vi "test bindata forth and back.vi"() -> ()   [LabVIEW 2018, in "LV-Julia_ZMQ-Roundtrip_lib.lvlib"]
uses:
  LV-Julia_ZMQ-Roundtrip_lib.lvlib
  05036e79-a137-49d8-b8bd-98c2707dfc19.vi
  d20d9b8d-18a0-4bcc-837d-245d5138e077.vi
  acfd4be8-0c55-499e-a24a-58fc6a9364d6.vi
  edd4ba47-7688-445c-9fb9-34873410a5b9.vi
  05036e79-a137-49d8-b8bd-98c2707dfc19.vi/236d3e0c-60a7-4ae5-9bc9-0ff41b983f05.vi
  05036e79-a137-49d8-b8bd-98c2707dfc19.vi/b449f9df-ee8d-489b-9487-897c21ba14eb.vi
  05036e79-a137-49d8-b8bd-98c2707dfc19.vi/e7b7674e-094d-4356-9454-cca6775f0358.vi
  05036e79-a137-49d8-b8bd-98c2707dfc19.vi/025d52f7-3b03-4309-bff2-4ec84fc3d60c.vi
  d20d9b8d-18a0-4bcc-837d-245d5138e077.vi/212a36f8-8f57-49c9-9677-432581b68510.vi
  d20d9b8d-18a0-4bcc-837d-245d5138e077.vi/69652d2b-db18-4aab-bd2f-35078bef0426.vi
  d20d9b8d-18a0-4bcc-837d-245d5138e077.vi/4772bca8-5d3a-4f2a-8bbf-c07de0696f94.vi
  d20d9b8d-18a0-4bcc-837d-245d5138e077.vi/7139aa7f-98bf-4369-975b-4bd5deaf00da.vi
  acfd4be8-0c55-499e-a24a-58fc6a9364d6.vi/b7780163-44f5-4435-ad3c-f5928cad1e22.vi
  acfd4be8-0c55-499e-a24a-58fc6a9364d6.vi/63841309-fb5d-4205-a56b-05074a2af6c9.vi
  edd4ba47-7688-445c-9fb9-34873410a5b9.vi/2b4cb753-bccd-455e-b921-2800034f5550.vi
  edd4ba47-7688-445c-9fb9-34873410a5b9.vi/9d483ba0-a828-48f7-8b88-1ec263ae9c55.vi
  05036e79-a137-49d8-b8bd-98c2707dfc19.vi/b449f9df-ee8d-489b-9487-897c21ba14eb.vi/9a929507-b059-4abd-9ed4-ef53a005ff63.vi
  05036e79-a137-49d8-b8bd-98c2707dfc19.vi/e7b7674e-094d-4356-9454-cca6775f0358.vi/ad73f5ce-7658-473b-b9fc-fac91a92da1e.vi
  05036e79-a137-49d8-b8bd-98c2707dfc19.vi/025d52f7-3b03-4309-bff2-4ec84fc3d60c.vi/5d27c3aa-c82a-4d9f-96ad-8781e4a71ba1.vi
  d20d9b8d-18a0-4bcc-837d-245d5138e077.vi/69652d2b-db18-4aab-bd2f-35078bef0426.vi/dfcf8de0-7860-4713-ab77-0e8f714dde10.vi
  d20d9b8d-18a0-4bcc-837d-245d5138e077.vi/4772bca8-5d3a-4f2a-8bbf-c07de0696f94.vi/e532232b-f4b6-4bbd-a5e7-664623875ae8.vi
  d20d9b8d-18a0-4bcc-837d-245d5138e077.vi/7139aa7f-98bf-4369-975b-4bd5deaf00da.vi/7a16f954-d622-4be0-bb4d-b4bfb8ef0f01.vi
  05036e79-a137-49d8-b8bd-98c2707dfc19.vi/b449f9df-ee8d-489b-9487-897c21ba14eb.vi/9a929507-b059-4abd-9ed4-ef53a005ff63.vi/47391a1c-e85f-44cf-90f5-ee97f4b4554e.vi
  05036e79-a137-49d8-b8bd-98c2707dfc19.vi/e7b7674e-094d-4356-9454-cca6775f0358.vi/ad73f5ce-7658-473b-b9fc-fac91a92da1e.vi/6213ee20-5898-4e73-9fb0-a99b3c67ea96.vi
  05036e79-a137-49d8-b8bd-98c2707dfc19.vi/025d52f7-3b03-4309-bff2-4ec84fc3d60c.vi/5d27c3aa-c82a-4d9f-96ad-8781e4a71ba1.vi/cb9fe9ca-b60f-4580-8939-faeac5c9a8ca.vi
  d20d9b8d-18a0-4bcc-837d-245d5138e077.vi/69652d2b-db18-4aab-bd2f-35078bef0426.vi/dfcf8de0-7860-4713-ab77-0e8f714dde10.vi/9577cbac-8520-44d1-a8fc-fc5a580fd613.vi
  d20d9b8d-18a0-4bcc-837d-245d5138e077.vi/4772bca8-5d3a-4f2a-8bbf-c07de0696f94.vi/e532232b-f4b6-4bbd-a5e7-664623875ae8.vi/9588a387-4c4f-45f1-904b-84c07455829b.vi
  d20d9b8d-18a0-4bcc-837d-245d5138e077.vi/7139aa7f-98bf-4369-975b-4bd5deaf00da.vi/7a16f954-d622-4be0-bb4d-b4bfb8ef0f01.vi/9c88b2f3-976e-4a83-96e4-93271b3fbf6a.vi
  05036e79-a137-49d8-b8bd-98c2707dfc19.vi/b449f9df-ee8d-489b-9487-897c21ba14eb.vi/9a929507-b059-4abd-9ed4-ef53a005ff63.vi/47391a1c-e85f-44cf-90f5-ee97f4b4554e.vi/32eb32a5-6c8c-4395-ad45-adfd19c3e226.vi
  05036e79-a137-49d8-b8bd-98c2707dfc19.vi/e7b7674e-094d-4356-9454-cca6775f0358.vi/ad73f5ce-7658-473b-b9fc-fac91a92da1e.vi/6213ee20-5898-4e73-9fb0-a99b3c67ea96.vi/ff21df5d-9d2e-4549-80bf-e7815593682d.vi
  05036e79-a137-49d8-b8bd-98c2707dfc19.vi/025d52f7-3b03-4309-bff2-4ec84fc3d60c.vi/5d27c3aa-c82a-4d9f-96ad-8781e4a71ba1.vi/cb9fe9ca-b60f-4580-8939-faeac5c9a8ca.vi/41816769-e1ec-46ec-9aae-7d6f9525b3ed.vi
  d20d9b8d-18a0-4bcc-837d-245d5138e077.vi/69652d2b-db18-4aab-bd2f-35078bef0426.vi/dfcf8de0-7860-4713-ab77-0e8f714dde10.vi/9577cbac-8520-44d1-a8fc-fc5a580fd613.vi/fbec7817-6f14-44c2-b008-b20ff5437b8a.vi
  d20d9b8d-18a0-4bcc-837d-245d5138e077.vi/4772bca8-5d3a-4f2a-8bbf-c07de0696f94.vi/e532232b-f4b6-4bbd-a5e7-664623875ae8.vi/9588a387-4c4f-45f1-904b-84c07455829b.vi/4f801452-6626-4e48-a8e0-47d2bc6ca629.vi
  d20d9b8d-18a0-4bcc-837d-245d5138e077.vi/7139aa7f-98bf-4369-975b-4bd5deaf00da.vi/7a16f954-d622-4be0-bb4d-b4bfb8ef0f01.vi/9c88b2f3-976e-4a83-96e4-93271b3fbf6a.vi/05c0184e-e222-4767-93e3-5fbdd5e0ae8f.vi
  check ID validity.vi
  <vilib>/Utility/error.llb/Error Cluster From Error Code.vi
panel:
  out "error out 2":errorcluster
  out "error out":errorcluster
  out "out 3D 2":dbl[][][](array[numeric]) format="%.2f"
  out "out 2D 2":dbl[][](array[numeric]) format="%.2f"
  out "out 1D 2":dbl[](array[numeric]) format="%.2f"
  out "arrdims":i32[](array[numeric])
  in  "dims0":u8=2 min=1 max=3
  in  "type0":i64
  out "sent 3D":dbl[][][](array[numeric])
  out "sent 2D":dbl[][](array[numeric])
  out "sent 1D":dbl[](array[numeric])
  out "out 1D":i64[](array[numeric])
  out "out 2D":i64[][](array[numeric])
  out "out 3D":i64[][][](array[numeric])
  in  "type1":dbl
  in  "dims1":u8=2 min=1 max=3
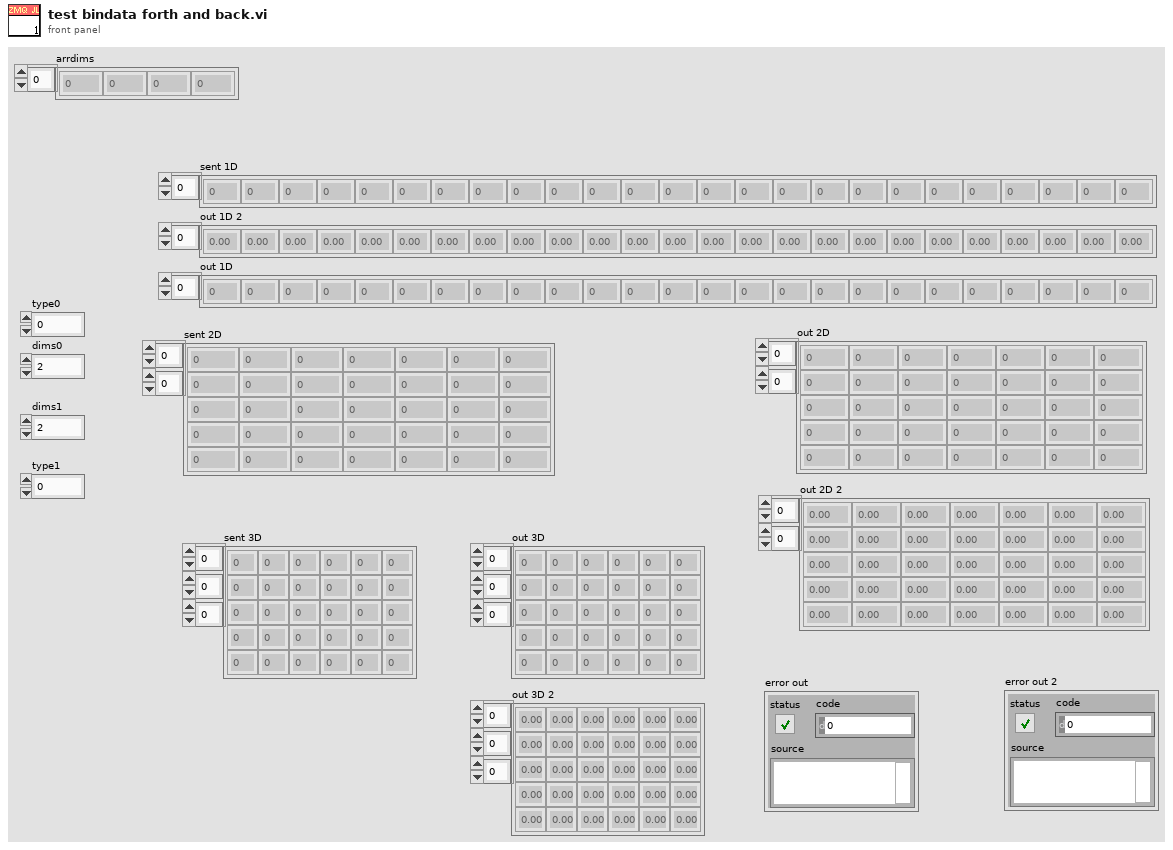
[diagram p1: front panel]
types:
  T1 = typedef "Bindata&description.ctl" = cluster{"bindata_descr":T2[], "bindata":u8[]}
  T2 = typedef "LV-Julia_ZMQ-Roundtrip_lib.lvlib/Bindata description.ctl" = cluster{"nofbytes":i32, "numtype":string, "start":i32, "arrdims":i32[], "kwarg_name":string, "category":string}
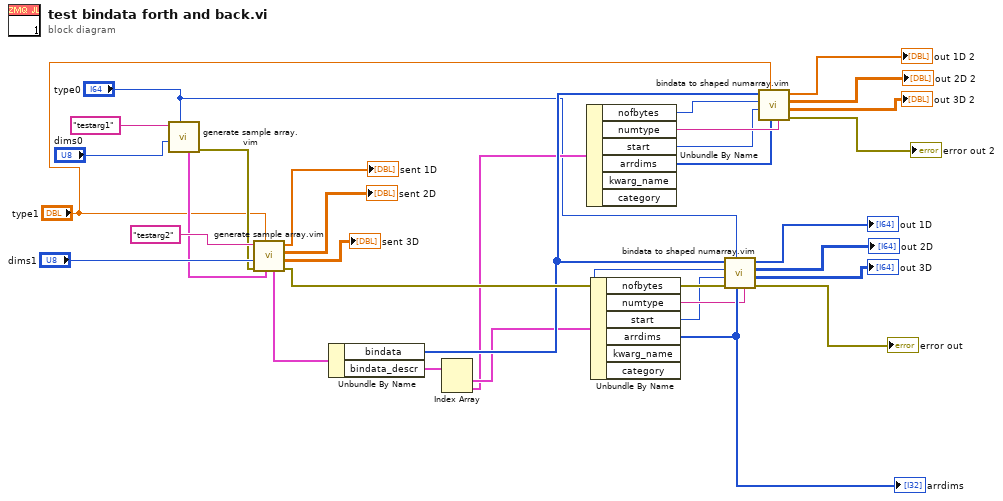
[diagram p0: block diagram]
diagram:
  n1 = call "generate sample array.vim"("type"="type0", "dims"="dims0", "kwarg_name"="testarg1") -> ("error out"=w18:errorcluster, "Bindata & descr out"=w19:T1)  [unwired: 3 in, 4 out]
  n2 = call "generate sample array.vim"("Bindata & descr in"=w19, "type"="type1", "error in (no error)"=w18, "dims"="dims1", "kwarg_name"="testarg2") -> ("error out"=w30:errorcluster, "Array 3D"=→"sent 3D":dbl[][][], "Array 2D"=→"sent 2D":dbl[][], "Array 1D"=→"sent 1D":dbl[], "Bindata & descr out"=w32:T1)  [unwired: 1 in, 1 out]
  n3 = Unbundle By Name(w32) -> ("bindata"=w11:u8[], "bindata_descr"=w31:T2[])
  n4 = Index Array(array=w31) -> (element #1=w4:T2, element #2=w3:T2)  [unwired: 2 in]
  n5 = Unbundle By Name(w3) -> ("nofbytes"=w10:i32, "numtype"=w9:string, "start"=w8:i32, "arrdims"=w7:i32[])  [unwired: 2 out]
  n6 = Unbundle By Name(w4) -> ("nofbytes"=w16:i32, "numtype"=w22:string, "start"=w15:i32, "arrdims"=w23:i32[])  [unwired: 2 out]
  "arrdims" <- w23
  n7 = call "bindata to shaped numarray.vim"("numtype in"=w22, "arrdims"=w23, "type in"="type0", "error in (no error)"=w30, "start"=w15, "nofbytes"=w16, "bindata in"=w11) -> ("error out"=→"error out":errorcluster, "numarray 3D"=→"out 3D":i64[][][], "numarray 2D"=→"out 2D":i64[][], "numarray 1D"=→"out 1D":i64[])  [unwired: 1 in]
  n8 = call "bindata to shaped numarray.vim"("numtype in"=w9, "arrdims"=w7, "type in"="type1", "start"=w8, "nofbytes"=w10, "bindata in"=w11) -> ("error out"=→"error out 2":errorcluster, "numarray 3D"=→"out 3D 2":dbl[][][], "numarray 2D"=→"out 2D 2":dbl[][], "numarray 1D"=→"out 1D 2":dbl[])  [unwired: 2 in]
